vi "get vi json graph description.vi"(8 "error in (no error)":errorcluster, 11 "vi path":string) -> (0 "error out":errorcluster, 2 "VI Description":string, 3 "JSON VI Graph":string)   [LabVIEW 2020]
doc: "**get vi json graph description.vi** opens a vi by path.\nIt scans recursively a VI's Block Diagram (including nested structures such as\nLoops and Case Structures) and returns a JSON object describing all objects,\ntheir wiring, and constant values. Output has four top-level array keys:\n\n\"0\" — Objects\n Every GObject found on the diagram: nodes, terminals, wires, diagrams,\n structures, constants.\n Fields: ClassID (LabVIEW internal class ID), UID (unique ref ID, valid\n for this scan only), ClassName (e.g. \"Function\", \"Wire\", \"Terminal\",\n \"ForLoop\", \"DigitalNumericConstant\"), LabelText (visible caption, if\n any), OwnerClass / OwnerName / Ownder_UID (immediate parent GObject).\n Note: \"Ownder_UID\" is a known typo in the field name, kept as-is for\n compatibility — do not treat it as an error.\n\n\"1\" — Wires (node-level)\n One entry per wire. UID_Wire (matches a \"Wire\" Object in array 0),\n UID_Source (owning-node UID of the wire's source terminal), UIDs_Sink\n (owning-node UID(s) of its sink terminal(s)). A wire may branch to\n multiple sinks; the same node UID can appear more than once if several\n of its terminals are fed by the same wire.\n\n\"2\" — Terminal-Wire mapping\n Resolves array \"1\" down to the exact terminal. Fields: \"Terminal UID\"\n (matches a Terminal-class Object in array 0), \"Wire UID\", \"Caption\"\n (the terminal's visible name/role, e.g. \"x\", \"output cluster\", \"x+1\";\n empty if the terminal has no visible caption).\n\n\"3\" — Constant values\n Fields: \"Constant UID\" (matches a *Constant-class Object in array 0),\n \"Value String\" (the constant's value as a JSON-formatted string). For\n ClusterConstant this is a full nested JSON object of all its fields.\n\nResolving a wire to its exact source/sink terminals:\n 1. Look up the wire in array \"1\" -> UID_Source, UIDs_Sink (node-level).\n 2. Find all entries in array \"2\" with matching \"Wire UID\" ? candidate\n terminal UIDs.\n 3. For each candidate, look up its Ownder_UID in array \"0\": if it\n equals UID_Source, that terminal is the source; if it appears in\n UIDs_Sink, it is a sink terminal.\n 4. Use \"Caption\" from array \"2\" for the terminal's semantic role\n (cluster field name, parameter name, etc.).\n\nKnown limitations:\n - Duplicate object entries may occasionally appear for the same UID\n (root cause not yet identified).\n - ClusterConstant \"Value String\" duplicates the values of its child\n constants (also listed individually) — provided as a convenience\n aggregate, not an independent value.\n - A constant's LabelText is a free-form caption; it is not necessarily\n related to the terminal/field it feeds."
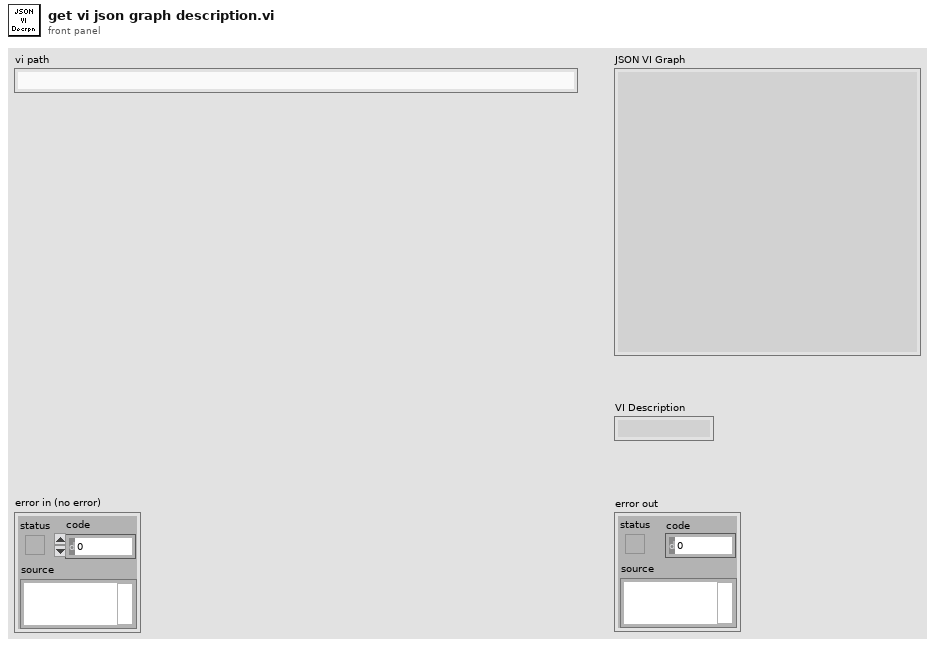
[diagram p1: front panel]
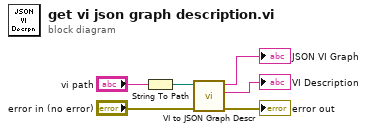
[diagram p0: block diagram]
diagram:
  n1 = String To Path(string="vi path") -> (path=w2:path)
  n2 = call "VI to JSON Graph Descr.vi"("error in (no error)"="error in (no error)", "vi path"=w2) -> ("error out"=→"error out":errorcluster, "VI Description"=→"VI Description":string, "JSON VI Graph"=→"JSON VI Graph":string)  [unwired: 7 in]
